vi "Set Colour.vi"(10 "Componant Colour":u32(colorbox), 11 "Game Componants in":refnum<class "Game Componants.lvclass">) -> (3 "Game Componants out":refnum<class "Game Componants.lvclass">)   [LabVIEW 2020, in "Game Componants.lvclass"]
uses:
  Game Componants.lvclass
  Game Componants.lvclass/Game Componants.ctl
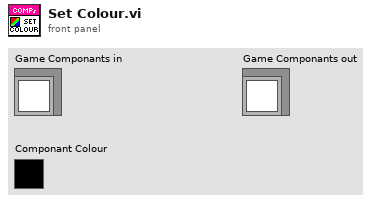
[diagram p1: front panel]
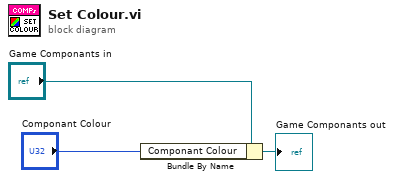
[diagram p0: block diagram]
diagram:
  n1 = Bundle By Name(cluster="Game Componants in", "Componant Colour"="Componant Colour") -> (→"Game Componants out":refnum<class "Game Componants.lvclass">)
